vi "MD5, Convert MD5 to DBL.vi"(5 "MD5":string="3da10dbfb34247d8b76754de4a8a0a76") -> (0 "MD5[0]":dbl=nan format="%.1f", 1 "MD5[1]":dbl=nan format="%.1f", 2 "MD5[2]":dbl=nan format="%.1f", 3 "MD5[3]":dbl=nan format="%.1f", 4 "int values":u32[](array[numeric]) format="%.0x")   [LabVIEW 2010]
doc: "This function converts four double precision floating point values into four unsigned 32-bit integers (8 hexadecimal digits) then concatenates the numbers into a single string (representing an MD5 message-digest).\n\nThe inverse of this function is \"MD5, Convert DBL to MD5.vi\""
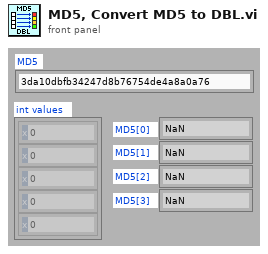
[diagram p1: front panel]
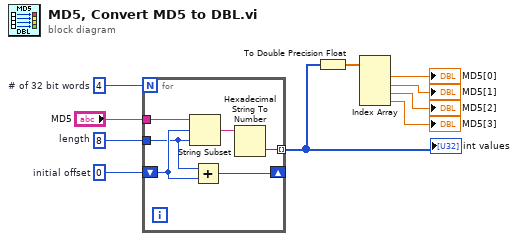
[diagram p0: block diagram]
diagram:
  w7 = 4  # # of 32 bit words
  w8 = 8  # length
  w9 = 0  # initial offset
  n1 = for {
    N: w7 -> [_]
    tunnel: "MD5" -> [w16]
    shift-right: [w14] -> _
    shift-left: w9 -> [w13]
    tunnel: w8 -> [w11]
    tunnel: [w12] -> w6 mode=indexing
    n2 = String Subset(string=w16, offset (0)=w13, length (rest)=w11) -> (substring=w15:string)
    n3 = Add(x=w11, y=w13) -> (x+y=w14:i32)
    n4 = Hexadecimal String To Number(string=w15) -> (number=w12:u32)  [unwired: 2 in, 1 out]
  }
  "int values" <- w6
  n5 = To Double Precision Float(number=w6) -> (double precision float=w5:dbl[])
  n6 = Index Array(array=w5) -> (element #1=→"MD5[0]":dbl, element #2=→"MD5[1]":dbl, element #3=→"MD5[2]":dbl, element #4=→"MD5[3]":dbl)  [unwired: 4 in]
